vi "Get Child Items.vi"(10 "Node":string, 11 "TreeControl in":refnum<vi>) -> (2 "Child Array":string[](array[string]), 3 "TreeControl out":refnum<vi>)   [LabVIEW 2021]
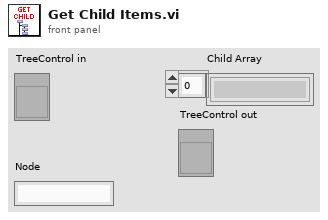
[diagram p1: front panel]
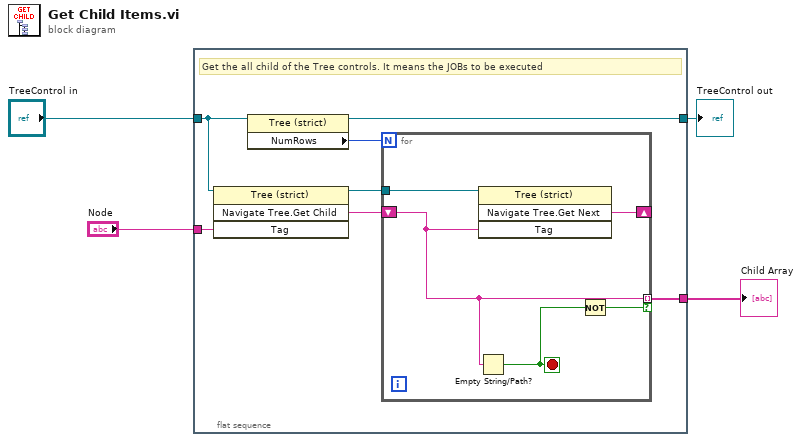
[diagram p0: block diagram]
diagram:
  n1 = flat-sequence {
    tunnel: [w10] -> w2
    tunnel: "Node" -> [w8]
    tunnel: "TreeControl in" -> [w6]
    tunnel: [w5] -> w1
    frame #0 {
      # "Get the all child of the Tree controls. It means the JOBs to be executed"
      n2 = invoke on="Invoke Node" class="Tree (strict)" method="Navigate Tree.Get Child"(reference=w6, "Tag"=w8) -> (reference out=w7:refnum<vi>, "Navigate Tree:Get Child"=w11:string)  [unwired: 2 in, 2 out]
      n3 = property on="Property Node" class="Tree (strict)"(reference=w6) -> (reference out=w5:refnum<vi>, "NumRows"=w9:u32)  [unwired: 1 in, 1 out]
      n4 = for {
        N: w9 -> [_]
        shift-right: [w16] -> _
        shift-left: w11 -> [w15]
        tunnel: [w15] -> w10 mode=indexing if=w13
        tunnel: w7 -> [w12]
        stop <- w14 stop-if-true
        n5 = Empty String/Path?(string/path=w15) -> (empty?=w14:bool)
        n6 = invoke on="Invoke Node" class="Tree (strict)" method="Navigate Tree.Get Next"(reference=w12, "Tag"=w15) -> ("Navigate Tree:Get Next Item"=w16:string)  [unwired: 2 in, 3 out]
        n7 = Not(x=w14) -> (.not. x?=w13:bool)
      }
    }
  }
  "Child Array" <- w2
  "TreeControl out" <- w1
